vi "Stop-Get.vi"(8 "error in (no error)":errorcluster, 11 "StopSignal Name(\"\" to use topmostVI)":string) -> (0 "error out":errorcluster, 1 "Stop?":bool, 2 "Reason":string, 3 "StopSignal":T1, 4 "timestamp":timestamp)   [LabVIEW 2020, in "StopSignal.lvlib"]
uses:
  StopSignal.lvlib
  Typedef/StopSignal.ctl
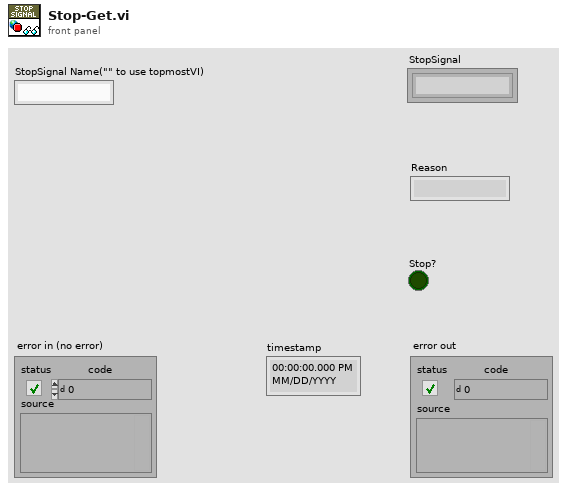
[diagram p1: front panel]
types:
  T1 = typedef "StopSignal.lvlib/StopSignal.ctl" = refnum<k1>
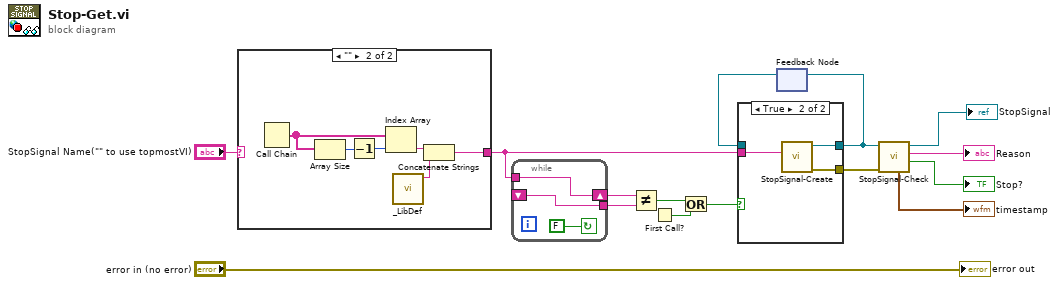
[diagram p0: block diagram]
diagram:
  n1 = case shown="\"\"" "StopSignal Name(\"\" to use topmostVI)" {
    selector: "StopSignal Name(\"\" to use topmostVI)" -> [w16 _]
    tunnel: [w16 w17] -> w2
    frame "False", Default {
    }
    frame "" {
      n2 = Call Chain() -> (call chain=w20:string[])
      n3 = Array Size(array=w20) -> (size(s)=w22:i32)
      n4 = Decrement(x=w22) -> (x-1=w21:i32)
      n5 = Index Array(array=w20, index=w21) -> (element=w19:string)
      n6 = call "_LibDef.vi"() -> ("LIBNAME"=w18:string)  [unwired: 11 in]
      n7 = Concatenate Strings(w19, w18) -> (w17:string)
    }
  }
  n8 = while {
    shift-right: [w25] -> w3
    shift-left: _ -> [w24]
    tunnel: w2 -> [w25]
    tunnel: [w24] -> w4
    stop <- FALSE continue-if-true
  }
  n9 = Not Equal?(x=w3, y=w4) -> (x != y?=w1:bool)
  n10 = First Call?() -> (First Call?: T/F=w10:bool)
  n11 = Or(x=w1, y=w10) -> (x .or. y?=w9:bool)
  n12 = feedback #1() -> (w8:T1)  [unwired: 1 in]
  n13 = case shown="True" w9 {
    tunnel: [_ w29] -> w15
    tunnel: [w26 w28] -> w11
    tunnel: w8 -> [w26 _]
    tunnel: w2 -> [_ w27]
    frame False {
    }
    frame True {
      n14 = call "StopSignal-Create.vi"("name(\"\")"=w27) -> ("error out"=w29:errorcluster, "StopSignal"=w28:T1)  [unwired: 9 in]
    }
  }
  n15 = feedback-in #1(w11) -> ()
  n16 = call "StopSignal-Check.vi"("error in (no error)"=w15, "StopSignal"=w11) -> ("Stop?"=→"Stop?":bool, "Reason"=→"Reason":string, "StopSignal(dup)"=→"StopSignal":T1, "timestamp"=→"timestamp":timestamp)  [unwired: 5 in, 1 out]
  "error out" <- "error in (no error)"
